vi "Inspect BBM Pad Groups.vi"(7 "Console Log in":refnum<class "Console Log.lvclass">, 8 "error in":errorcluster, 10 "Module Data In":T1={"TBM-TBM"={"Fiducial Image"={"Image Position"=refnum, "Image Reference"=refnum, "Field of View"={"x(mm)"=0.0, "y(mm)"=0.0}}, "Fiducials"=[]}, "TBM-HDI"={"Fiducial Image"={"Image Position"=refnum, "Image Reference"=refnum, "Field of View"={"x(mm)"=0.0, "y(mm)"=0.0}}, "Fiducials"=[]}, "Address Pads"={"Fiducial Image"={"Image Position"=refnum, "Image Reference"=refnum, "Field of View"={"x(mm)"=0.0, "y(mm)"=0.0}}, "Fiducials"=[]}, "HDI Bond Pad References"=[], "BBM Bond Pad References"=[], "HV-HDI"={"Fiducial Image"={"Image Position"=refnum, "Image Reference"=refnum, "Field of View"={"x(mm)"=0.0, "y(mm)"=0.0}}, "Selected Fiducial"={"Fiducial Image Coordinate"=refnum, "Fiducial Source"=enum."Pattern Recognition"}, "fiducial name"=""}, "HV-BBM"={"Fiducial Image"={"Image Position"=refnum, "Image Reference"=refnum, "Field of View"={"x(mm)"=0.0, "y(mm)"=0.0}}, "Selected Fiducial"={"Fiducial Image Coordinate"=refnum, "Fiducial Source"=enum."Pattern Recognition"}, "fiducial name"=""}, "Chuck"=0, "Slot"=0, "Potting Selection"={"HDI Bond Pads"=[TRUE, TRUE, TRUE, TRUE, TRUE, TRUE, TRUE, TRUE, TRUE, TRUE, TRUE, TRUE, TRUE, TRUE, TRUE, TRUE], "BBM Bond Pads"=[TRUE, TRUE, TRUE, TRUE, TRUE, TRUE, TRUE, TRUE, TRUE, TRUE, TRUE, TRUE, TRUE, TRUE, TRUE, TRUE], "TBM Inner"={"Top"=TRUE, "Left"=TRUE, "Bottom"=TRUE, "Right"=TRUE}, "TBM Outer"={"Top"=TRUE, "Left"=TRUE, "Bottom"=TRUE, "Right"=TRUE}, "Address Pads"={"Top"=TRUE, "Bottom"=TRUE}, "High Voltage"={"HDI"=TRUE, "BBM"=TRUE}}}, 11 "Potting Procedure in":refnum<class "Potting Procedure.lvclass">) -> (0 "error out":errorcluster, 2 "Module Data Out":T1={"TBM-TBM"={"Fiducial Image"={"Image Position"=refnum, "Image Reference"=refnum, "Field of View"={"x(mm)"=0.0, "y(mm)"=0.0}}, "Fiducials"=[]}, "TBM-HDI"={"Fiducial Image"={"Image Position"=refnum, "Image Reference"=refnum, "Field of View"={"x(mm)"=0.0, "y(mm)"=0.0}}, "Fiducials"=[]}, "Address Pads"={"Fiducial Image"={"Image Position"=refnum, "Image Reference"=refnum, "Field of View"={"x(mm)"=0.0, "y(mm)"=0.0}}, "Fiducials"=[]}, "HDI Bond Pad References"=[], "BBM Bond Pad References"=[], "HV-HDI"={"Fiducial Image"={"Image Position"=refnum, "Image Reference"=refnum, "Field of View"={"x(mm)"=0.0, "y(mm)"=0.0}}, "Selected Fiducial"={"Fiducial Image Coordinate"=refnum, "Fiducial Source"=enum."Pattern Recognition"}, "fiducial name"=""}, "HV-BBM"={"Fiducial Image"={"Image Position"=refnum, "Image Reference"=refnum, "Field of View"={"x(mm)"=0.0, "y(mm)"=0.0}}, "Selected Fiducial"={"Fiducial Image Coordinate"=refnum, "Fiducial Source"=enum."Pattern Recognition"}, "fiducial name"=""}, "Chuck"=0, "Slot"=0, "Potting Selection"={"HDI Bond Pads"=[TRUE, TRUE, TRUE, TRUE, TRUE, TRUE, TRUE, TRUE, TRUE, TRUE, TRUE, TRUE, TRUE, TRUE, TRUE, TRUE], "BBM Bond Pads"=[TRUE, TRUE, TRUE, TRUE, TRUE, TRUE, TRUE, TRUE, TRUE, TRUE, TRUE, TRUE, TRUE, TRUE, TRUE, TRUE], "TBM Inner"={"Top"=TRUE, "Left"=TRUE, "Bottom"=TRUE, "Right"=TRUE}, "TBM Outer"={"Top"=TRUE, "Left"=TRUE, "Bottom"=TRUE, "Right"=TRUE}, "Address Pads"={"Top"=TRUE, "Bottom"=TRUE}, "High Voltage"={"HDI"=TRUE, "BBM"=TRUE}}}, 3 "Potting Procedure out":refnum<class "Potting Procedure.lvclass">, 5 "Console Log out":refnum<class "Console Log.lvclass">)   [LabVIEW 2011, in "Potting Procedure.lvclass"]
uses:
  Potting Procedure.lvclass
  Application Utilities/Console Log/Console Log.lvclass
  Type Definitions/Inspect Modules - Module.ctl
  Shared Components/Vec3d Class/Vec3d Class.lvclass
  Shared Components/Utils/Type Definitions/Multi-Fiducial Image.ctl
  Shared Components/Utils/Type Definitions/Physical Image.ctl
  <vilib>/vision/Image Controls.llb/IMAQ Image.ctl
  Shared Components/Utils/Type Definitions/Fiducial with Source.ctl
  Shared Components/Utils/Type Definitions/Fiducial Image.ctl
  Shared Components/WorkTable Class/WorkTable Class.lvclass
  Shared Components/Gantry Class/Gantry Class.lvclass
  Shared Components/Config Manager Class/Type Definitions/Camera Enum.ctl
  Shared Components/Config Manager Class/Type Definitions/Part Type.ctl
  Shared Components/Config Manager Class/Read Geometry Definition 3D.vi
  Shared Components/Config Manager Class/Config Manager Class.lvclass
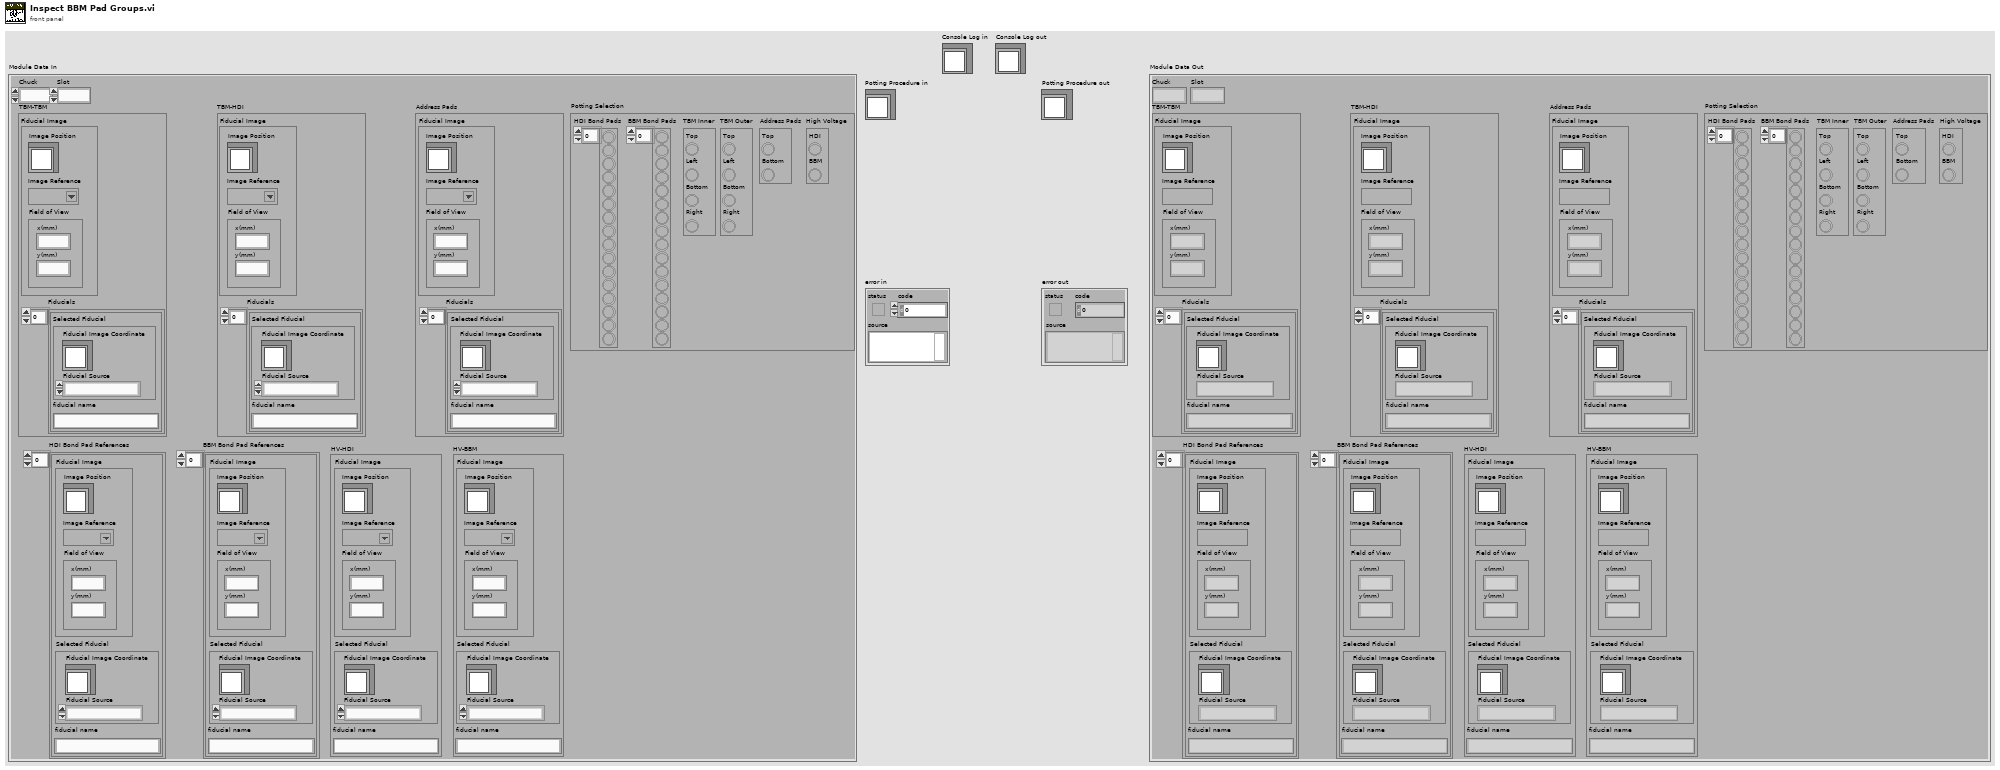
[diagram p1: front panel]
types:
  T1 = typedef "Inspect Modules - Module.ctl" = cluster{"TBM-TBM":T2, "TBM-HDI":T2, "Address Pads":T2, "HDI Bond Pad References":T6[], "BBM Bond Pad References":T6[], "HV-HDI":T6, "HV-BBM":T6, "Chuck":i32, "Slot":i32, "Potting Selection":cluster{"HDI Bond Pads":bool[], "BBM Bond Pads":bool[], "TBM Inner":cluster{"Top":bool, "Left":bool, "Bottom":bool, "Right":bool}, "TBM Outer":cluster{"Top":bool, "Left":bool, "Bottom":bool, "Right":bool}, "Address Pads":cluster{"Top":bool, "Bottom":bool}, "High Voltage":cluster{"HDI":bool, "BBM":bool}}}
  T2 = typedef "Multi-Fiducial Image.ctl" = cluster{"Fiducial Image":T3, "Fiducials":cluster{"Selected Fiducial":T5, "fiducial name":string}[]}
  T3 = typedef "Physical Image.ctl" = cluster{"Image Position":refnum<class "Vec3d Class.lvclass">, "Image Reference":T4, "Field of View":cluster{"x(mm)":dbl, "y(mm)":dbl}}
  T4 = typedef "IMAQ Image.ctl" = refnum<image>
  T5 = typedef "Fiducial with Source.ctl" = cluster{"Fiducial Image Coordinate":refnum<class "Vec3d Class.lvclass">, "Fiducial Source":enum16{"Pattern Recognition", "User", "Error", "Default"}}
  T6 = typedef "Fiducial Image.ctl" = cluster{"Fiducial Image":T3, "Selected Fiducial":T5, "fiducial name":string}
  T7 = typedef "Camera Enum.ctl" = enum16{"GANTRY HEAD", "NEEDLE CALIBRATION X", "NEEDLE CALIBRATION Y"}
  T8 = typedef "Part Type.ctl" = enum16{"BBM", "HDI", "BARE HDI", "GLUERESERVOIR", "STAMP_1", "STAMP_2", "STAMP_3", "STAMP_4", "STAMP_5", "WEIGHT_1", "WEIGHT_2", "WEIGHT_3", "WEIGHT_4", "WEIGHT_5", "WEIGHT_6", "WEIGHT_7", "WEIGHT_8", "PICKER_TOOL", "GRABER_TOOL"}
  T9 = enum16{"Pattern Recognition", "User", "Error", "Default"}
  T10 = typedef "Worktable_Module Slot.ctl" = cluster{"Slot State":enum16{"Empty", "Bare HDI", "Unglued", "Stamped", "PartOnTop", "Weighted", "Unpotted", "Potted"}, "BBM Type":enum16{"None", "BBM", "GlassSlide"}, "HDI Type":enum16{"None", "HDI", "Polyimide"}, "Vacuum Channel":u8, "Location/Orientation BBM":T11, "Location/Orientation HDI":T11, "S/N":string}
  T11 = typedef "Position_Orientation.ctl" = cluster{"Center":refnum<class "Vec3d Class.lvclass">, "Orientation":refnum<class "Orient3d Class.lvclass">}
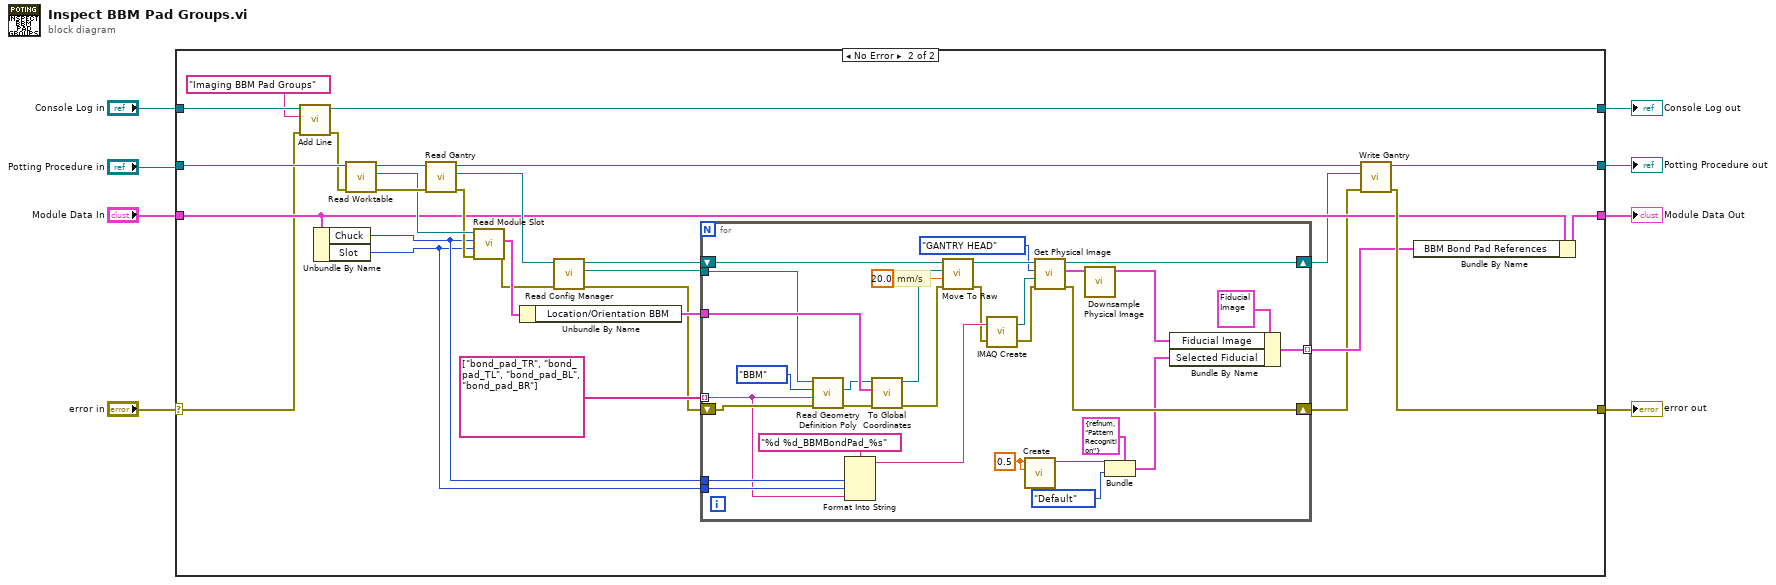
[diagram p0: block diagram]
diagram:
  n1 = case shown="No Error" "error in" {
    selector: "error in" -> [w11 w14]
    tunnel: [w11 w29] -> w6
    tunnel: [w12 w30] -> w5
    tunnel: "Potting Procedure in" -> [w12 w40]
    tunnel: "Module Data In" -> [w10 w28]
    tunnel: [w10 w32] -> w1
    tunnel: "Console Log in" -> [w9 w27]
    tunnel: [w9 w25] -> w3
    frame Error {
    }
    frame No Error {
      n2 = call "Add Line.vi"("error in"=w14, "String"="Imaging BBM Pad Groups", "Console Log in"=w27) -> ("error out"=w13:errorcluster, "Console Log out"=w25:refnum<class "Console Log.lvclass">)  [unwired: 7 in]
      n3 = Unbundle By Name(w28) -> ("Chuck"=w20:i32, "Slot"=w19:i32)
      n4 = call-dynamic "Read Worktable.vi"("error in"=w13, "Potting Procedure in"=w40) -> ("error out"=w38:errorcluster, "WorkTable out"=w37:refnum<class "WorkTable Class.lvclass">, "Potting Procedure out"=w39:refnum<class "Potting Procedure.lvclass">)  [unwired: 7 in]
      n5 = call-dynamic "Read Gantry.vi"("error in (no error)"=w38, "Potting Procedure in"=w39) -> ("error out"=w36:errorcluster, "Gantry"=w34:refnum<class "Gantry Class.lvclass">, "Potting Procedure out"=w31:refnum<class "Potting Procedure.lvclass">)  [unwired: 7 in]
      n6 = call-dynamic "Read Module Slot.vi"("error in"=w36, "slot"=w19, "chuck"=w20, "WorkTable in"=w37) -> ("error out"=w33:errorcluster, "Module Slot"=w35:T10)  [unwired: 5 in, 1 out]
      n7 = Unbundle By Name(w35) -> ("Location/Orientation BBM"=w22:T11)
      n8 = call-dynamic "Read Config Manager.vi"("error in"=w33, "Gantry in"=w34) -> ("error out"=w15:errorcluster, "Config Manager"=w23:refnum<class "Config Manager Class.lvclass">, "Gantry out"=w24:refnum<class "Gantry Class.lvclass">)  [unwired: 7 in]
      n9 = for {
        tunnel: string[] ["bond_pad_TR", "bond_pad_TL", "bond_pad_BL", "bond_pad_BR"] -> [w46] mode=indexing
        tunnel: w22 -> [w71]
        shift-right: [w57] -> w17
        shift-left: w15 -> [w47]
        tunnel: w20 -> [w64]
        tunnel: w19 -> [w63]
        shift-right: [w58] -> w16
        shift-left: w24 -> [w70]
        tunnel: [w50] -> w18 mode=indexing
        tunnel: w23 -> [w49]
        w52 = 0.5 ("X")
        # "mm/s"
        n10 = call-poly "Read Geometry Definition Poly.vi"("error in"=w47, "Feature"=w46, "Part Type"=Part_Type."BBM", "Config Manager in"=w49) -> ("error out"=w44:errorcluster, "Feature Coordinates"=w45:refnum<class "Vec3d Class.lvclass">)  [unwired: 5 in, 1 out]
        n11 = Format Into String(format string="%d %d_BBMBondPad_%s", w64, w63, w46) -> (resulting string=w62:string)  [unwired: 2 in, 1 out]
        n12 = call "To Global Coordinates.vi"("error in"=w44, "Center/Orientation"=w71, "Local Coordinates"=w45) -> ("error out"=w67:errorcluster, "Global Coordinates"=w69:refnum<class "Vec3d Class.lvclass">)  [unwired: 7 in]
        n13 = call-dynamic "Move To Raw.vi"("error in"=w67, "Speed"=20.0, "Destination"=w69, "Gantry in"=w70) -> ("error out"=w61:errorcluster, "Gantry out"=w66:refnum<class "Gantry Class.lvclass">)  [unwired: 6 in]
        n14 = call "IMAQ Create"("Image Name"=w62, "error in (no error)"=w61) -> ("New Image"=w59:T4, "error out"=w60:errorcluster)  [unwired: 3 in]
        n15 = call "Create.vi"("Y"=w52, "X"=w52) -> ("Vec3d Class out"=w53:refnum<class "Vec3d Class.lvclass">)  [unwired: 8 in, 1 out]
        n16 = call-dynamic "Get Physical Image.vi"("error in"=w60, "Image In"=w59, "Camera Name"=Camera_Enum."GANTRY HEAD", "Gantry in"=w66) -> ("error out"=w57:errorcluster, "Physical Image"=w42:T3, "Gantry out"=w58:refnum<class "Gantry Class.lvclass">)  [unwired: 5 in]
        n17 = call "Downsample Physical Image.vi"("Physical Image In"=w42) -> ("Physical Image Out"=w41:T3)  [unwired: 9 in, 1 out]
        n18 = Bundle(cluster=T5 {"Fiducial Image Coordinate"=refnum, "Fiducial Source"=enum."Pattern Recognition"} ("Selected Fiducial"), "Fiducial Image Coordinate"=w53, "Fiducial Source"=T9."Default") -> (w54:T5)
        n19 = Bundle By Name(cluster=T6 {"Fiducial Image"={"Image Position"=refnum, "Image Reference"=refnum, "Field of View"={"x(mm)"=0.0, "y(mm)"=0.0}}, "Selected Fiducial"={"Fiducial Image Coordinate"=refnum, "Fiducial Source"=enum."Pattern Recognition"}, "fiducial name"=""} ("Fiducial Image"), "Fiducial Image"=w41, "Selected Fiducial"=w54) -> (w50:T6)
      }
      n20 = call-dynamic "Write Gantry.vi"("error in (no error)"=w17, "Gantry"=w16, "Potting Procedure in"=w31) -> ("error out"=w29:errorcluster, "Potting Procedure out"=w30:refnum<class "Potting Procedure.lvclass">)  [unwired: 7 in]
      n21 = Bundle By Name(cluster=w28, "BBM Bond Pad References"=w18) -> (w32:T1)
    }
  }
  "error out" <- w6
  "Potting Procedure out" <- w5
  "Console Log out" <- w3
  "Module Data Out" <- w1
